vi "AccelerationBrakeDetect.vi"(5 "油门1输入":dbl format="%#_16g", 6 "油门2输入":dbl format="%#_16g", 7 "刹车输入":dbl format="%#_16g") -> (0 "油门1":dbl format="%#_16g", 1 "油门2":dbl format="%#_16g", 2 "刹车":dbl format="%#_616g", 3 "上次运行有故障？":bool, 4 "Implausibility":bool=TRUE)   [LabVIEW 2013]
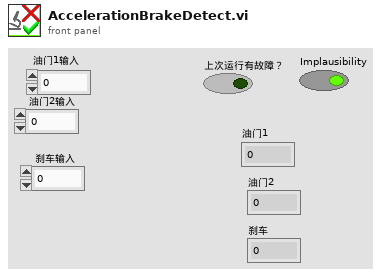
[diagram p1: front panel]
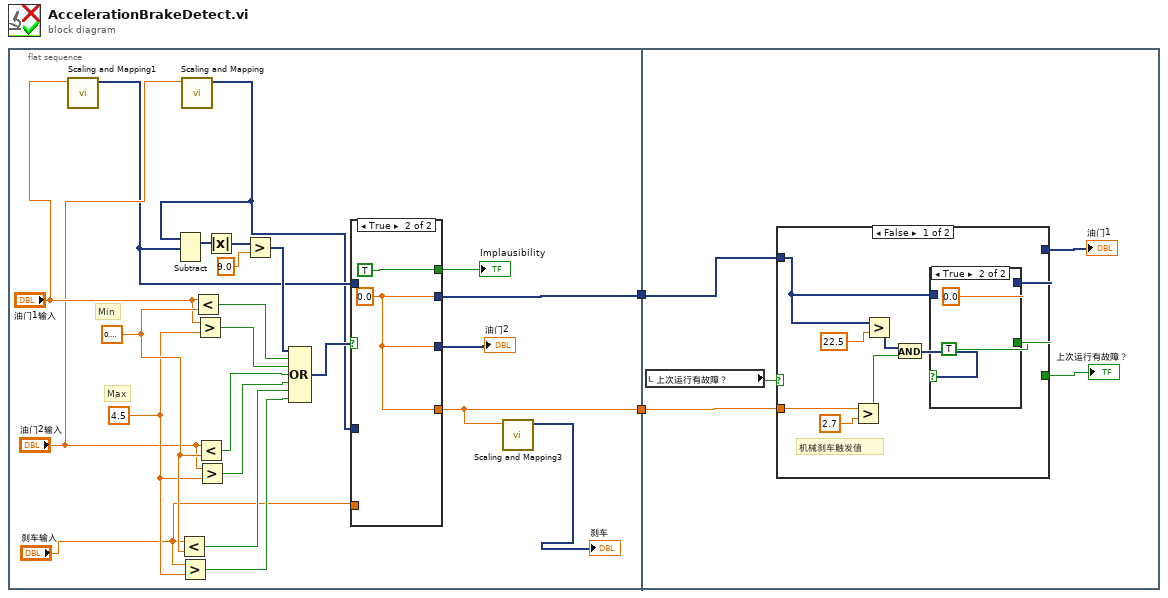
[diagram p0: block diagram]
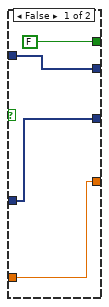
[diagram p2: hidden frame]
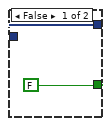
[diagram p3: hidden frame]
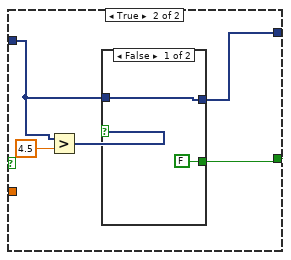
[diagram p4: hidden frame]
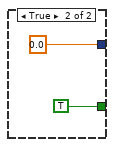
[diagram p5: hidden frame]
diagram:
  n1 = flat-sequence {
    tunnel: [w23] -> w2
    tunnel: [w4] -> w1
    tunnel: w2 -> [w36]
    tunnel: w1 -> [w34]
    frame #0 {
      w14 = sgl 4.5 ("y")
      w15 = sgl 0.4 ("y")
      # "Min"
      # "Max"
      n2 = call "Scaling and Mapping1"("Signals"="油门1输入") -> ("Scaled Signals"=w6:dynamicdata)  [unwired: 9 in, 1 out]
      n3 = Less?(x="刹车输入", y=w15) -> (x < y?=w17:bool)
      n4 = Greater?(x="刹车输入", y=w14) -> (0:w16:bool)
      n5 = call "Scaling and Mapping"("Signals"="油门2输入") -> ("Scaled Signals"=w5:dynamicdata)  [unwired: 9 in, 1 out]
      n6 = Subtract(1:w6, 2:w5) -> (0:w25:dynamicdata)  [unwired: 1 in, 1 out]
      n7 = Less?(x="油门1输入", y=w15) -> (x < y?=w21:bool)
      n8 = Greater?(x="油门1输入", y=w14) -> (0:w20:bool)
      n9 = Less?(x="油门2输入", y=w15) -> (x < y?=w19:bool)
      n10 = Greater?(x="油门2输入", y=w14) -> (0:w18:bool)
      n11 = Absolute Value(x=w25) -> (abs(x)=w8:dynamicdata)
      n12 = Greater?(x=w8, y=9.0) -> (0:w7:dynamicdata)
      n13 = Compound Arithmetic op=OR(w7, w21, w20, w19, w18, w17, w16) -> (w22:dynamicdata)
      n14 = case shown="True" w22 {
        tunnel: [w29 w31] -> w23
        tunnel: [w26 w31] -> w13
        tunnel: [w27 w31] -> w4
        tunnel: w6 -> [w29 _]
        tunnel: w5 -> [w26 _]
        tunnel: "刹车输入" -> [w27 _]
        tunnel: [FALSE TRUE] -> w11
        frame False {
        }
        frame True {
          w31 = 0.0
        }
      }
      "Implausibility" <- w11
      "油门2" <- w13
      n15 = call "Scaling and Mapping3"("Signals"=w4) -> ("Scaled Signals"=→"刹车":dynamicdata)  [unwired: 9 in, 1 out]
    }
    frame #1 {
      n16 = local read "上次运行有故障？"() -> (w33:bool)
      n17 = case shown="False" w33 {
        tunnel: w36 -> [w38 w50]
        tunnel: [w41 w52] -> w35
        tunnel: w34 -> [w40 _]
        tunnel: [w39 w51] -> w32
        frame False {
          # "机械刹车触发值"
          n18 = Greater?(x=w40, y=2.7) -> (0:w43:bool)
          n19 = Greater?(x=w38, y=22.5) -> (0:w44:dynamicdata)
          n20 = And(x=w44, y=w43) -> (x .and. y?=w42:dynamicdata)
          n21 = case shown="True" w42 {
            tunnel: w38 -> [w47 _]
            tunnel: [w47 0.0 ("油门1")] -> w41
            tunnel: [FALSE ("上次运行有故障？") TRUE ("上次运行有故障？")] -> w39
            frame False {
            }
            frame True {
            }
          }
        }
        frame True {
          n22 = Greater?(x=w50, y=4.5) -> (0:w53:dynamicdata)
          n23 = case shown="False" w53 {
            tunnel: [w56 0.0 ("油门1")] -> w52
            tunnel: w50 -> [w56 _]
            tunnel: [FALSE ("上次运行有故障？") TRUE ("上次运行有故障？")] -> w51
            frame False {
            }
            frame True {
            }
          }
        }
      }
      "油门1" <- w35
      "上次运行有故障？" <- w32
    }
  }
